vi "Master Setup Read Write RT Setup Strings.vi"(8 "error in (no error)":errorcluster, 9 "Read (F)/Write (T)":bool, 10 "Pattern Label":T1 items=["Channel Setup (0)", "PID Setup (1)", "Filter Setup (2)", "~Reserved Old CAN Msgs (3)", "~Reserved Old CAN1 (4)", "~Reserved Old CAN2 (5)", "Digital Inputs Setup (6)", "Digital Outputs Setup (7)", "Logging 1 Setup (8)", "Logging 2 Setup (9)", "Logging 3 Setup (10)", "Setpoint Setup (11)", "Test Series Setup (12)", "Graph Setup (13)", "System Configure (14)", "Header (15)", "Profile Manager (16)", "Post-Mortem Logging (17)", "High-Speed Data (18)", "Statistic Channel Setup (19)", "Ramp Channel Setup (20)", "ETAS INCA Channel Setup (21)", "ETC ECCS Transducer Setup (22)", "ETC ECCS Test Setup (23)", "AVL AK Smoke Meter Setup (24)", "Triggers Setup (25)", "Alarm Limits Setup (26)", "YKWT1 Measurement (27)", "YKWT1 Instrument (28)", "Auto File Settings (29)", "Playback File Setting (30)", "UUT Constants (31)", "UPS Setup (32)", "Differential Channel Setup (33)", "Integral Channel Setup (34)", "Signal Channel Setup (35)", "Calibration Setup (36)", "BNC Setup (37)", "ASAP3 Setup (38)", "Chassis Force Calculations (39)", "Chassis Teststand Losses (40)", "Chassis Vehicle Losses (41)", "Formula Channels (42)", "ASAP3 Map Coords Setup (43)", "Digital Controls Setup (44)", "Push Buttons Setup (45)", "Sliders Setup (46)", "~Reserved~ (47)", "Email Setup (48)", "Timer Setup (49)", "Unit Conversion Setup (50)", "Visible Channels (51)", "Main Display Setup (52)", "Message Display Setup (53)", "Input Display Setup (54)", "Unico Parameter Downloads (55)", "Flow Meter Setup (56)", "Channel Zero Offset (57)", "YKWT2 Measurement (58)", "YKWT2 Instrument (59)", "~Reserved Old CAN3 (60)", "CAS Setup (61)", "Accumulation Channel Setup (62)", "Valvetrain Dynamics Setup (63)", "CCP Setup (64)", "System Log Setup (65)", "Throttle Controller (66)", "RE Shifter (67)", "Main Display (68)", "~Reserved~ (69)", "FlexRay (70)", "YKWT3 Measurement (71)", "YKWT3 Instrument (72)", "CAN XNET API (73)"], 11 "RT Setup String (in)":string) -> (0 "error out":errorcluster, 3 "RT Setup String (out)":string)   [LabVIEW 2017]
uses:
  Master Setup Pattern Enum.ctl
panel:
  in  "Setup File (System Configure)":path=path "C:/Revolutionary Engineering/REPS/Setup Files/Default/GM Trans Cell 2/SystemConfigure GM cell 2.cfs"
  in  "Setup File (Setpoint)":path=path "C:/Revolutionary Engineering/REPS/Setup Files/Default/RE Cell 3-1/re cell 3 setpoints.spt"
  in  "Setup File (CAN 0)":path
  in  "Setup File (CAN 1)":path
  in  "Setup File (Can Message)":path
  in  "Setup File (Playback)":path
  in  "Setup File (UUT Constants)":path
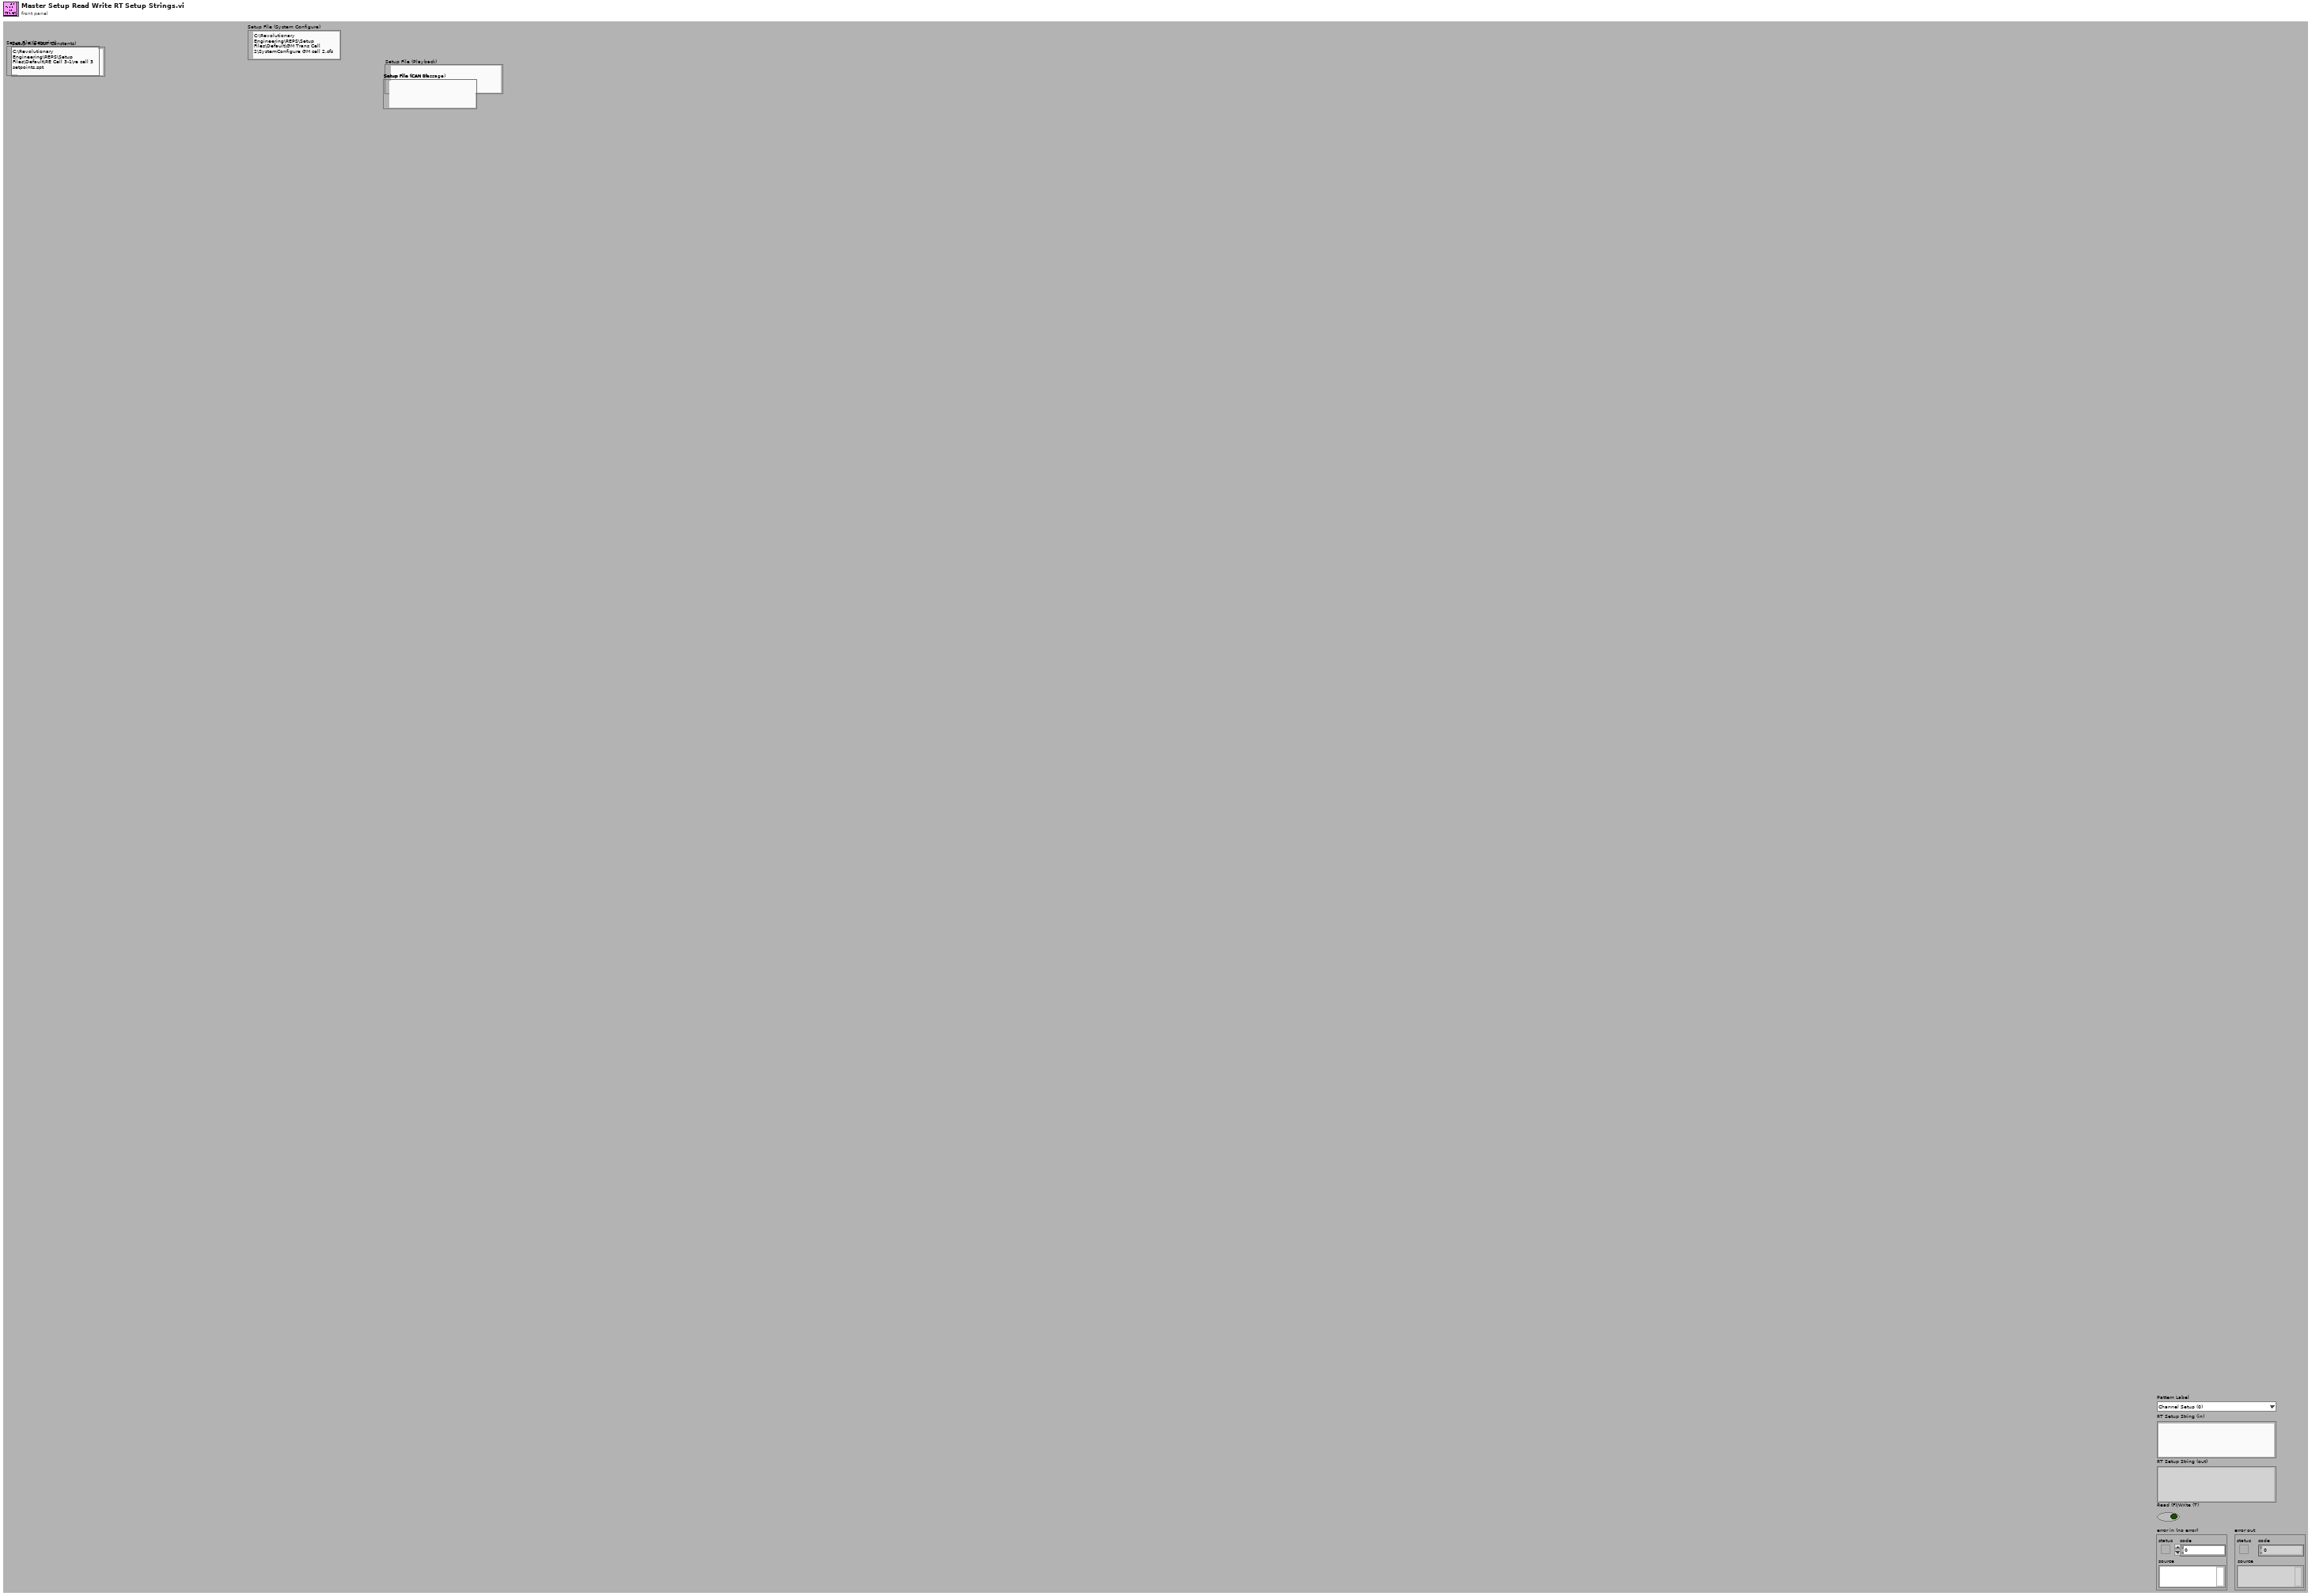
[diagram p1: front panel]
types:
  T1 = typedef "Master Setup Pattern Enum.ctl" = i32
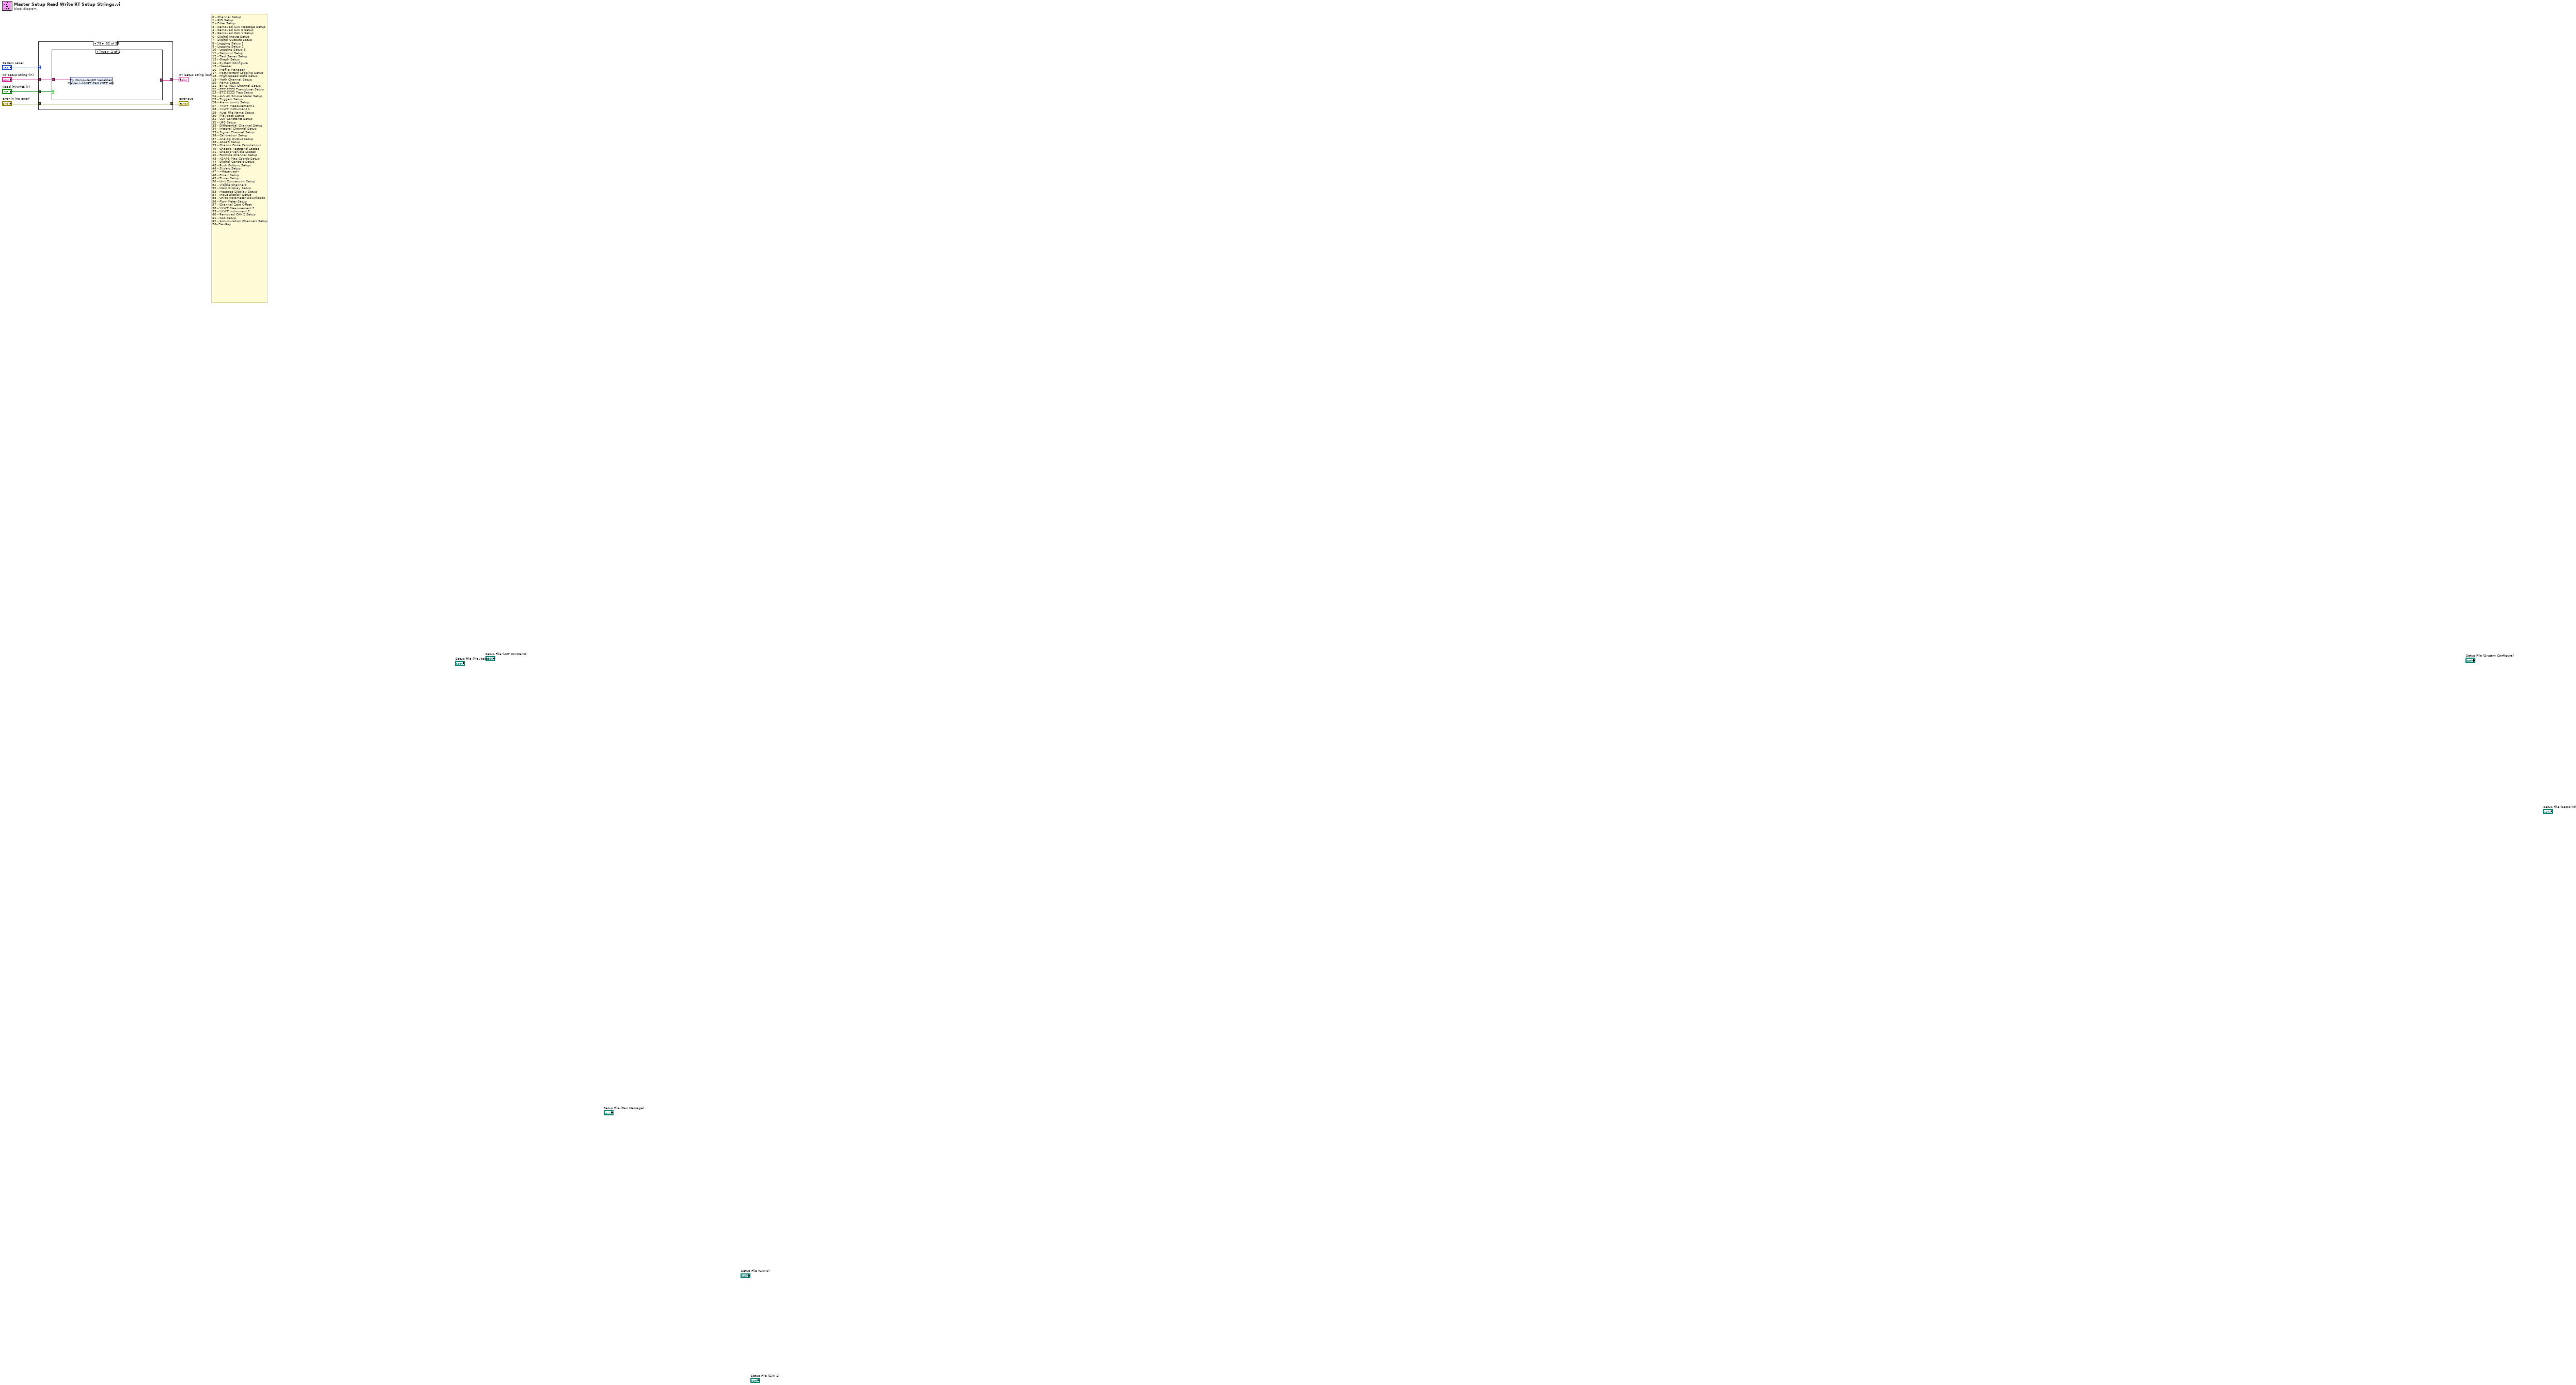
[diagram p0: block diagram]
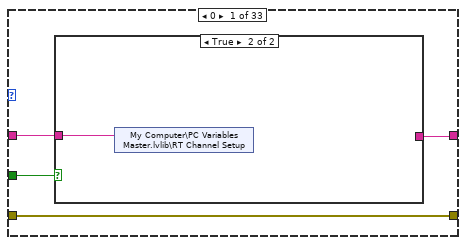
[diagram p2: hidden frame]
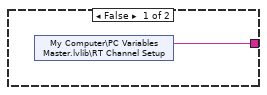
[diagram p3: hidden frame]
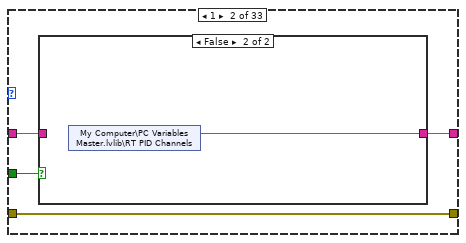
[diagram p4: hidden frame]
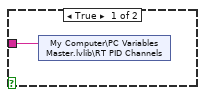
[diagram p5: hidden frame]
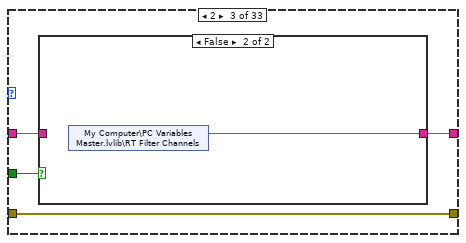
[diagram p6: hidden frame]
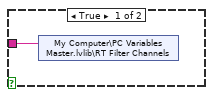
[diagram p7: hidden frame]
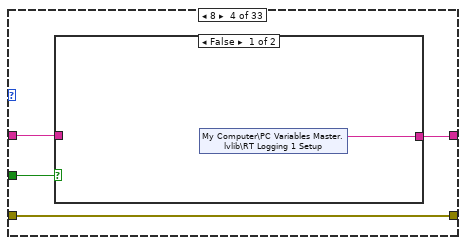
[diagram p8: hidden frame]
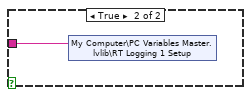
[diagram p9: hidden frame]
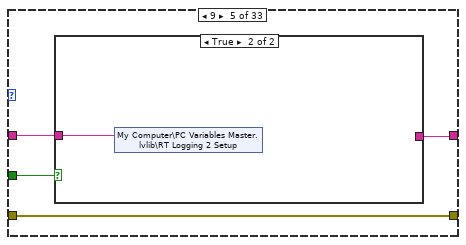
[diagram p10: hidden frame]
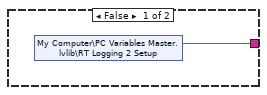
[diagram p11: hidden frame]
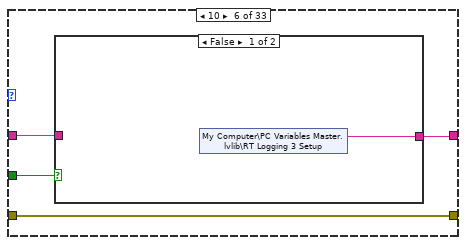
[diagram p12: hidden frame]
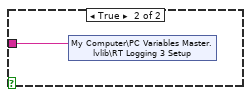
[diagram p13: hidden frame]
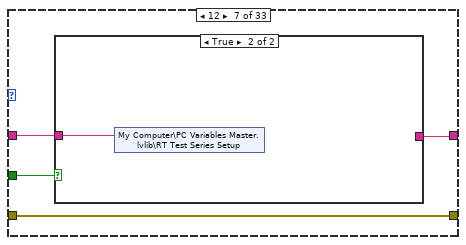
[diagram p14: hidden frame]
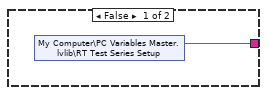
[diagram p15: hidden frame]
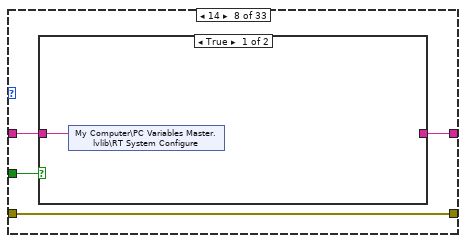
[diagram p16: hidden frame]
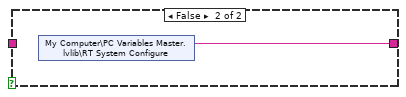
[diagram p17: hidden frame]
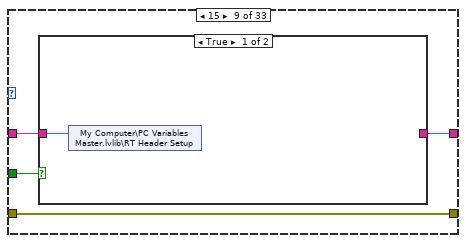
[diagram p18: hidden frame]
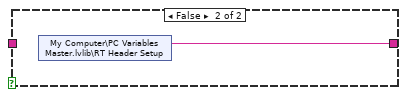
[diagram p19: hidden frame]
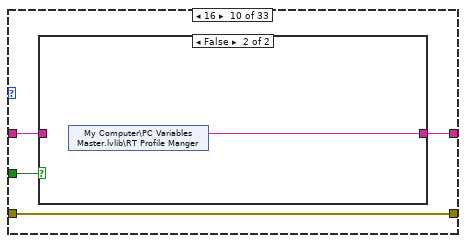
[diagram p20: hidden frame]
diagram:
  # "0 - Channel Setup\n1 - PID Setup\n2 - Filter Setup\n3 - Removed CAN Message Setup\n4 - Removed CAN 0 Setup\n5 - Removed CAN 1 Setup\n6 - Digital Inputs Setup\n7 - Digital Outputs Setup\n8 - Logging Setup 1\n9 - Logging Setup 2\n10 - Logging Setup 3\n11 - Setpoint Setup\n12 - Test Series Setup\n13 - Graph Setup\n14 - System Configure\n15 - Header\n16 - Profile Manager\n17 - Post-Mortem Logging Setup\n18 - High-Speed Data Setup\n19 - Math Channel Setup\n20 - Ramp Setup\n21 - ETAS INCA Channel Setup\n22 - ETC ECCS Transducer Setup\n23 - ETC ECCS Test Setup\n24 - AVL AK Smoke Meter Setup\n25 - Triggers Setup\n26 - Alarm Limits Setup\n27 - YKWT Measurement 1\n28 - YKWT Instrument 1\n29 - Auto File Name Setup\n30 - Playback Setup\n31 - UUT Constants Setup\n32 - UPS Setup\n33 - Differential Channel Setup\n34 - Integral Channel Setup\n35 - Signal Channel Setup\n36 - Calibration Setup\n37 - Analog Output Setup\n38 - ASAP3 Setup\n39 - Chassis Force Calculations\n40 - Chassis Teststand Losses\n41 - Chassis Vehicle Losses\n42 - Formula Channel Setup\n43 - ASAP3 Map Coords Setup\n44 - Digital Controls Setup\n45 - Push Buttons Setup\n46 - Sliders Setup\n47 - ~Reserved~\n48 - Email Setup\n49 - Timer Setup\n50 - Unit Conversion Setup\n51 - Visible Channels\n52 - Main Display Setup\n53 - Message Display Setup\n54 - Input Display Setup\n55 - Unico Parameter Downloads\n56 - Flow Meter Setup\n57 - Channel Zero Offset\n58 - YKWT Measurement 2\n59 - YKWT Instrument 2\n60 - Removed CAN 2 Setup\n61 - CAS Setup\n62 - Accumulation Channels Setup\n70- FlexRay"
  n1 = case shown="73" "Pattern Label" {
    tunnel: "Read (F)/Write (T)" -> [w10 w16 w22 w28 w34 w40 w46 w52 w58 w64 w70 w76 w82 w88 w94 w100 w106 w112 w118 w124 w130 w136 w142 w148 w154 w159 w166 w172 w178 w184 w190 w196 _]
    tunnel: "RT Setup String (in)" -> [w8 w15 w21 w26 w32 w38 w44 w51 w57 w63 w69 w75 w81 w87 w92 w99 w105 w111 w117 w122 w128 w135 w141 w147 w153 w158 w164 w170 w176 w182 w188 w194 _]
    tunnel: [w9 w14 w20 w27 w33 w39 w45 w50 w56 w62 w68 w74 w80 w86 w93 w98 w104 w110 w116 w123 w129 w134 w140 w146 w152 w157 w165 w171 w177 w183 w189 w195 _] -> w3
    tunnel: "error in (no error)" -> [w7 w13 w19 w25 w31 w37 w43 w49 w55 w61 w67 w73 w79 w85 w91 w97 w103 w109 w115 w121 w127 w133 w139 w145 w151 w160 w163 w169 w175 w181 w187 w193 w200]
    tunnel: [w7 w13 w19 w25 w31 w37 w43 w49 w55 w61 w67 w73 w79 w85 w91 w97 w103 w109 w115 w121 w127 w133 w139 w145 w151 w160 w163 w169 w175 w181 w187 w193 w199] -> w1
    frame 0 {
      n2 = case shown="True" w10 {
        tunnel: [w11 _] -> w9
        tunnel: w8 -> [_ w12]
        frame False {
          n3 = shared-variable "My Computer\\PC Variables Master.lvlib\\RT Channel Setup"() -> (w11:string)  [unwired: 1 in, 1 out]
        }
        frame True {
          n4 = shared-variable "My Computer\\PC Variables Master.lvlib\\RT Channel Setup"(w12) -> ()  [unwired: 1 in, 1 out]
        }
      }
    }
    frame 1 {
      n5 = case shown="False" w16 {
        tunnel: w15 -> [w17 _]
        tunnel: [_ w18] -> w14
        frame True {
          n6 = shared-variable "My Computer\\PC Variables Master.lvlib\\RT PID Channels"(w17) -> ()  [unwired: 1 in, 1 out]
        }
        frame False {
          n7 = shared-variable "My Computer\\PC Variables Master.lvlib\\RT PID Channels"() -> (w18:string)  [unwired: 1 in, 1 out]
        }
      }
    }
    frame 2 {
      n8 = case shown="False" w22 {
        tunnel: w21 -> [w23 _]
        tunnel: [_ w24] -> w20
        frame True {
          n9 = shared-variable "My Computer\\PC Variables Master.lvlib\\RT Filter Channels"(w23) -> ()  [unwired: 1 in, 1 out]
        }
        frame False {
          n10 = shared-variable "My Computer\\PC Variables Master.lvlib\\RT Filter Channels"() -> (w24:string)  [unwired: 1 in, 1 out]
        }
      }
    }
    frame 8 {
      n11 = case shown="False" w28 {
        tunnel: [w29 _] -> w27
        tunnel: w26 -> [_ w30]
        frame False {
          n12 = shared-variable "My Computer\\PC Variables Master.lvlib\\RT Logging 1 Setup"() -> (w29:string)  [unwired: 1 in, 1 out]
        }
        frame True {
          n13 = shared-variable "My Computer\\PC Variables Master.lvlib\\RT Logging 1 Setup"(w30) -> ()  [unwired: 1 in, 1 out]
        }
      }
    }
    frame 9 {
      n14 = case shown="True" w34 {
        tunnel: [w35 _] -> w33
        tunnel: w32 -> [_ w36]
        frame False {
          n15 = shared-variable "My Computer\\PC Variables Master.lvlib\\RT Logging 2 Setup"() -> (w35:string)  [unwired: 1 in, 1 out]
        }
        frame True {
          n16 = shared-variable "My Computer\\PC Variables Master.lvlib\\RT Logging 2 Setup"(w36) -> ()  [unwired: 1 in, 1 out]
        }
      }
    }
    frame 10 {
      n17 = case shown="False" w40 {
        tunnel: [w41 _] -> w39
        tunnel: w38 -> [_ w42]
        frame False {
          n18 = shared-variable "My Computer\\PC Variables Master.lvlib\\RT Logging 3 Setup"() -> (w41:string)  [unwired: 1 in, 1 out]
        }
        frame True {
          n19 = shared-variable "My Computer\\PC Variables Master.lvlib\\RT Logging 3 Setup"(w42) -> ()  [unwired: 1 in, 1 out]
        }
      }
    }
    frame 12 {
      n20 = case shown="True" w46 {
        tunnel: [w47 _] -> w45
        tunnel: w44 -> [_ w48]
        frame False {
          n21 = shared-variable "My Computer\\PC Variables Master.lvlib\\RT Test Series Setup"() -> (w47:string)  [unwired: 1 in, 1 out]
        }
        frame True {
          n22 = shared-variable "My Computer\\PC Variables Master.lvlib\\RT Test Series Setup"(w48) -> ()  [unwired: 1 in, 1 out]
        }
      }
    }
    frame 14 {
      n23 = case shown="True" w52 {
        tunnel: w51 -> [w53 _]
        tunnel: [_ w54] -> w50
        frame True {
          n24 = shared-variable "My Computer\\PC Variables Master.lvlib\\RT System Configure"(w53) -> ()  [unwired: 1 in, 1 out]
        }
        frame False {
          n25 = shared-variable "My Computer\\PC Variables Master.lvlib\\RT System Configure"() -> (w54:string)  [unwired: 1 in, 1 out]
        }
      }
    }
    frame 15 {
      n26 = case shown="True" w58 {
        tunnel: w57 -> [w59 _]
        tunnel: [_ w60] -> w56
        frame True {
          n27 = shared-variable "My Computer\\PC Variables Master.lvlib\\RT Header Setup"(w59) -> ()  [unwired: 1 in, 1 out]
        }
        frame False {
          n28 = shared-variable "My Computer\\PC Variables Master.lvlib\\RT Header Setup"() -> (w60:string)  [unwired: 1 in, 1 out]
        }
      }
    }
    frame 16 {
      n29 = case shown="False" w64 {
        tunnel: w63 -> [w65 _]
        tunnel: [_ w66] -> w62
        frame True {
          n30 = shared-variable "My Computer\\PC Variables Master.lvlib\\RT Profile Manger"(w65) -> ()  [unwired: 1 in, 1 out]
        }
        frame False {
          n31 = shared-variable "My Computer\\PC Variables Master.lvlib\\RT Profile Manger"() -> (w66:string)  [unwired: 1 in, 1 out]
        }
      }
    }
    frame 17 {
      n32 = case shown="True" w70 {
        tunnel: w69 -> [w71 _]
        tunnel: [_ w72] -> w68
        frame True {
          n33 = shared-variable "My Computer\\PC Variables Master.lvlib\\RT Logging PM Setup"(w71) -> ()  [unwired: 1 in, 1 out]
        }
        frame False {
          n34 = shared-variable "My Computer\\PC Variables Master.lvlib\\RT Logging PM Setup"() -> (w72:string)  [unwired: 1 in, 1 out]
        }
      }
    }
    frame 19 {
      n35 = case shown="False" w76 {
        tunnel: w75 -> [w77 _]
        tunnel: [_ w78] -> w74
        frame True {
          n36 = shared-variable "My Computer\\PC Variables Master.lvlib\\RT Math Channels"(w77) -> ()  [unwired: 1 in, 1 out]
        }
        frame False {
          n37 = shared-variable "My Computer\\PC Variables Master.lvlib\\RT Math Channels"() -> (w78:string)  [unwired: 1 in, 1 out]
        }
      }
    }
    frame 20 {
      n38 = case shown="True" w82 {
        tunnel: w81 -> [w83 _]
        tunnel: [_ w84] -> w80
        frame True {
          n39 = shared-variable "My Computer\\PC Variables Master.lvlib\\RT Ramp Channels"(w83) -> ()  [unwired: 1 in, 1 out]
        }
        frame False {
          n40 = shared-variable "My Computer\\PC Variables Master.lvlib\\RT Ramp Channels"() -> (w84:string)  [unwired: 1 in, 1 out]
        }
      }
    }
    frame 25 {
      n41 = case shown="True" w88 {
        tunnel: w87 -> [w89 _]
        tunnel: [_ w90] -> w86
        frame True {
          n42 = shared-variable "My Computer\\PC Variables Master.lvlib\\RT Trigger Channels"(w89) -> ()  [unwired: 1 in, 1 out]
        }
        frame False {
          n43 = shared-variable "My Computer\\PC Variables Master.lvlib\\RT Trigger Channels"() -> (w90:string)  [unwired: 1 in, 1 out]
        }
      }
    }
    frame 26 {
      n44 = case shown="True" w94 {
        tunnel: [w95 _] -> w93
        tunnel: w92 -> [_ w96]
        frame False {
          n45 = shared-variable "My Computer\\PC Variables Master.lvlib\\RT Alarm Limits Setup"() -> (w95:string)  [unwired: 1 in, 1 out]
        }
        frame True {
          n46 = shared-variable "My Computer\\PC Variables Master.lvlib\\RT Alarm Limits Setup"(w96) -> ()  [unwired: 1 in, 1 out]
        }
      }
    }
    frame 30 {
      n47 = case shown="True" w100 {
        tunnel: w99 -> [w101 _]
        tunnel: [_ w102] -> w98
        frame True {
          n48 = shared-variable "My Computer\\PC Variables Master.lvlib\\RT Playback Setup"(w101) -> ()  [unwired: 1 in, 1 out]
        }
        frame False {
          n49 = shared-variable "My Computer\\PC Variables Master.lvlib\\RT Playback Setup"() -> (w102:string)  [unwired: 1 in, 1 out]
        }
      }
    }
    frame 33 {
      n50 = case shown="True" w106 {
        tunnel: w105 -> [w107 _]
        tunnel: [_ w108] -> w104
        frame True {
          n51 = shared-variable "My Computer\\PC Variables Master.lvlib\\RT Differential Channels"(w107) -> ()  [unwired: 1 in, 1 out]
        }
        frame False {
          n52 = shared-variable "My Computer\\PC Variables Master.lvlib\\RT Differential Channels"() -> (w108:string)  [unwired: 1 in, 1 out]
        }
      }
    }
    frame 34 {
      n53 = case shown="True" w112 {
        tunnel: w111 -> [w113 _]
        tunnel: [_ w114] -> w110
        frame True {
          n54 = shared-variable "My Computer\\PC Variables Master.lvlib\\RT Integration Channels"(w113) -> ()  [unwired: 1 in, 1 out]
        }
        frame False {
          n55 = shared-variable "My Computer\\PC Variables Master.lvlib\\RT Integration Channels"() -> (w114:string)  [unwired: 1 in, 1 out]
        }
      }
    }
    frame 35 {
      n56 = case shown="True" w118 {
        tunnel: w117 -> [w119 _]
        tunnel: [_ w120] -> w116
        frame True {
          n57 = shared-variable "My Computer\\PC Variables Master.lvlib\\RT Waveform Signal Channels"(w119) -> ()  [unwired: 1 in, 1 out]
        }
        frame False {
          n58 = shared-variable "My Computer\\PC Variables Master.lvlib\\RT Waveform Signal Channels"() -> (w120:string)  [unwired: 1 in, 1 out]
        }
      }
    }
    frame 36 {
      n59 = case shown="True" w124 {
        tunnel: [w125 _] -> w123
        tunnel: w122 -> [_ w126]
        frame False {
          n60 = shared-variable "My Computer\\PC Variables Master.lvlib\\RT Calibration Setup"() -> (w125:string)  [unwired: 1 in, 1 out]
        }
        frame True {
          n61 = shared-variable "My Computer\\PC Variables Master.lvlib\\RT Calibration Setup"(w126) -> ()  [unwired: 1 in, 1 out]
        }
      }
    }
    frame 37 {
      n62 = case shown="False" w130 {
        tunnel: [w131 _] -> w129
        tunnel: w128 -> [_ w132]
        frame False {
          n63 = shared-variable "My Computer\\PC Variables Master.lvlib\\RT BNC Setup"() -> (w131:string)  [unwired: 1 in, 1 out]
        }
        frame True {
          n64 = shared-variable "My Computer\\PC Variables Master.lvlib\\RT BNC Setup"(w132) -> ()  [unwired: 1 in, 1 out]
        }
      }
    }
    frame 42 {
      n65 = case shown="False" w136 {
        tunnel: w135 -> [w137 _]
        tunnel: [_ w138] -> w134
        frame True {
          n66 = shared-variable "My Computer\\PC Variables Master.lvlib\\RT Formula Channels"(w137) -> ()  [unwired: 1 in, 1 out]
        }
        frame False {
          n67 = shared-variable "My Computer\\PC Variables Master.lvlib\\RT Formula Channels"() -> (w138:string)  [unwired: 1 in, 1 out]
        }
      }
    }
    frame 45 {
      n68 = case shown="True" w142 {
        tunnel: w141 -> [w143 _]
        tunnel: [_ w144] -> w140
        frame True {
          n69 = shared-variable "My Computer\\PC Variables Master.lvlib\\RT Push Button Setup"(w143) -> ()  [unwired: 1 in, 1 out]
        }
        frame False {
          n70 = shared-variable "My Computer\\PC Variables Master.lvlib\\RT Push Button Setup"() -> (w144:string)  [unwired: 1 in, 1 out]
        }
      }
    }
    frame 49 {
      n71 = case shown="False" w148 {
        tunnel: w147 -> [_ w150]
        tunnel: [w149 _] -> w146
        frame False {
          n72 = shared-variable "My Computer\\PC Variables Master.lvlib\\RT Timer Channels"() -> (w149:string)  [unwired: 1 in, 1 out]
        }
        frame True {
          n73 = shared-variable "My Computer\\PC Variables Master.lvlib\\RT Timer Channels"(w150) -> ()  [unwired: 1 in, 1 out]
        }
      }
    }
    frame 50 {
      n74 = case shown="True" w154 {
        tunnel: w153 -> [w155 _]
        tunnel: [_ w156] -> w152
        frame True {
          n75 = shared-variable "My Computer\\PC Variables Master.lvlib\\RT Unit Conversion"(w155) -> ()  [unwired: 1 in, 1 out]
        }
        frame False {
          n76 = shared-variable "My Computer\\PC Variables Master.lvlib\\RT Unit Conversion"() -> (w156:string)  [unwired: 1 in, 1 out]
        }
      }
    }
    frame 56 {
      n77 = case shown="False" w159 {
        tunnel: w158 -> [_ w162]
        tunnel: [w161 _] -> w157
        frame False {
          n78 = shared-variable "My Computer\\PC Variables Master.lvlib\\RT Flow Meter Channels"() -> (w161:string)  [unwired: 1 in, 1 out]
        }
        frame True {
          n79 = shared-variable "My Computer\\PC Variables Master.lvlib\\RT Flow Meter Channels"(w162) -> ()  [unwired: 1 in, 1 out]
        }
      }
    }
    frame 57 {
      n80 = case shown="True" w166 {
        tunnel: [w167 _] -> w165
        tunnel: w164 -> [_ w168]
        frame False {
          n81 = shared-variable "My Computer\\PC Variables Master.lvlib\\RT Zero Offset Setup"() -> (w167:string)  [unwired: 1 in, 1 out]
        }
        frame True {
          n82 = shared-variable "My Computer\\PC Variables Master.lvlib\\RT Zero Offset Setup"(w168) -> ()  [unwired: 1 in, 1 out]
        }
      }
    }
    frame 62 {
      n83 = case shown="False" w172 {
        tunnel: [w173 _] -> w171
        tunnel: w170 -> [_ w174]
        frame False {
          n84 = shared-variable "My Computer\\PC Variables Master.lvlib\\RT Accumulation Channels"() -> (w173:string)  [unwired: 1 in, 1 out]
        }
        frame True {
          n85 = shared-variable "My Computer\\PC Variables Master.lvlib\\RT Accumulation Channels"(w174) -> ()  [unwired: 1 in, 1 out]
        }
      }
    }
    frame 65 {
      n86 = case shown="False" w178 {
        tunnel: [w179 _] -> w177
        tunnel: w176 -> [_ w180]
        frame False {
          n87 = shared-variable "My Computer\\PC Variables Master.lvlib\\RT System log Setup"() -> (w179:string)  [unwired: 1 in, 1 out]
        }
        frame True {
          n88 = shared-variable "My Computer\\PC Variables Master.lvlib\\RT System log Setup"(w180) -> ()  [unwired: 1 in, 1 out]
        }
      }
    }
    frame 64 {
      n89 = case shown="True" w184 {
        tunnel: [w185 _] -> w183
        tunnel: w182 -> [_ w186]
        frame False {
          n90 = shared-variable "My Computer\\PC Variables Master.lvlib\\RT CCP Setup"() -> (w185:string)  [unwired: 1 in, 1 out]
        }
        frame True {
          n91 = shared-variable "My Computer\\PC Variables Master.lvlib\\RT CCP Setup"(w186) -> ()  [unwired: 1 in, 1 out]
        }
      }
    }
    frame 70 {
      n92 = case shown="False" w190 {
        tunnel: [w191 _] -> w189
        tunnel: w188 -> [_ w192]
        frame False {
          n93 = shared-variable "My Computer\\PC Variables Master.lvlib\\RT FlexRay"() -> (w191:string)  [unwired: 1 in, 1 out]
        }
        frame True {
          n94 = shared-variable "My Computer\\PC Variables Master.lvlib\\RT FlexRay"(w192) -> ()  [unwired: 1 in, 1 out]
        }
      }
    }
    frame 73 {
      n95 = case shown="True" w196 {
        tunnel: [w197 _] -> w195
        tunnel: w194 -> [_ w198]
        frame False {
          n96 = shared-variable "My Computer\\PC Variables Master.lvlib\\RT CAN XNET API"() -> (w197:string)  [unwired: 1 in, 1 out]
        }
        frame True {
          n97 = shared-variable "My Computer\\PC Variables Master.lvlib\\RT CAN XNET API"(w198) -> ()  [unwired: 1 in, 1 out]
        }
      }
    }
    frame Default {
      n98 = Select(t=w200, s=w200, f=errorcluster {"status"=TRUE, "code"=0, "source"=""}) -> (s? t:f=w199:errorcluster)
    }
  }
  "RT Setup String (out)" <- w3
  "error out" <- w1
